vi "Write XML Node.vi"(6 "attributes":T1[](array[typedef]), 8 "error in (no error)":errorcluster, 9 "body":string, 10 "node":string, 11 "initial string":string) -> (0 "error out":errorcluster, 3 "resulting string":string)   [LabVIEW 2020, in "XMLGen.lvlib"]
uses:
  <vilib>/AppBuilder/Engine/WebServiceDescription/XMLGen/XMLGen.lvlib
  <vilib>/AppBuilder/Engine/WebServiceDescription/XMLGen/ValuePair.ctl
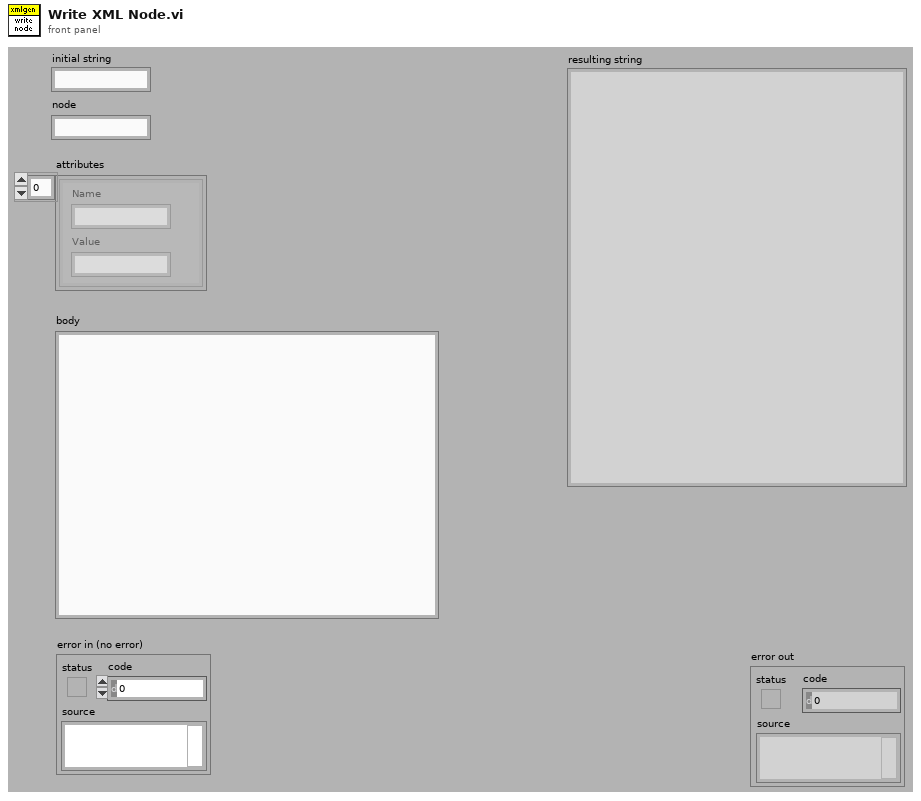
[diagram p1: front panel]
types:
  T1 = typedef "XMLGen.lvlib/ValuePair.ctl" = cluster{"Name":string, "Value":string}
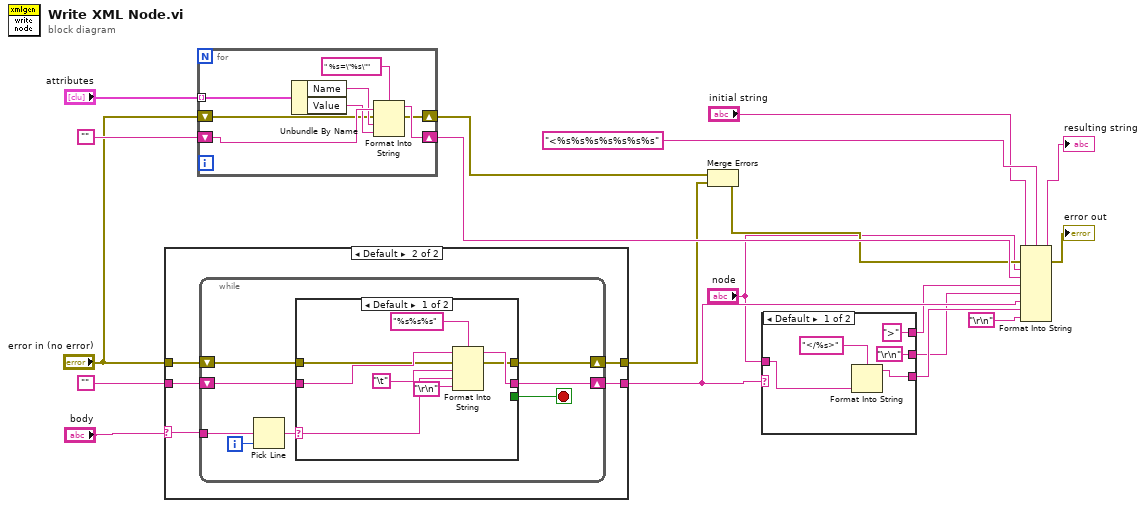
[diagram p0: block diagram]
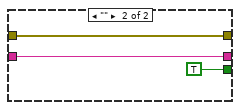
[diagram p3: hidden frame]
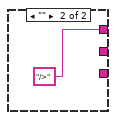
[diagram p4: hidden frame]
diagram:
  n1 = case shown="Default" "body" {
    selector: "body" -> [w21 w22]
    tunnel: "" -> [_ w26]
    tunnel: "error in (no error)" -> [w20 w25]
    tunnel: [w20 w24] -> w12
    tunnel: [w21 w23] -> w5
    frame "" {
    }
    frame Default {
      n2 = while {
        shift-right: [w29] -> w23
        shift-left: w26 -> [w30]
        tunnel: w22 -> [w33]
        shift-right: [w27] -> w24
        shift-left: w25 -> [w28]
        i -> [w34]
        stop <- w31 stop-if-true
        n3 = Pick Line(multi-line string=w33, line index=w34) -> (output string=w32:string)  [unwired: 1 out]
        n4 = case shown="Default" w32 {
          selector: w32 -> [w41 _]
          tunnel: [_ TRUE] -> w31
          tunnel: [w38 w45] -> w29
          tunnel: w30 -> [w42 w45]
          tunnel: w28 -> [w37 w44]
          tunnel: [w36 w44] -> w27
          frame Default {
            n5 = Format Into String(format string="%s%s%s", initial string=w42, error in=w37, "\t", w41, "\r\n") -> (resulting string=w38:string, error out=w36:errorcluster)
          }
          frame "" {
          }
        }
      }
    }
  }
  n6 = for {
    tunnel: "attributes" -> [w51] mode=indexing
    shift-right: [w48] -> w16
    shift-left: "" -> [w53]
    shift-right: [w46] -> w13
    shift-left: "error in (no error)" -> [w47]
    n7 = Unbundle By Name(w51) -> ("Name"=w50:string, "Value"=w49:string)
    n8 = Format Into String(format string=" %s=\"%s\"", initial string=w53, error in=w47, w50, w49) -> (resulting string=w48:string, error out=w46:errorcluster)
  }
  n9 = Merge Errors(w13, w12) -> (w11:errorcluster)
  n10 = case shown="Default" w5 {
    tunnel: [w58 _] -> w6
    tunnel: "node" -> [w56 _]
    tunnel: [">" "/>"] -> w2
    tunnel: ["\r\n" _] -> w1
    frame Default {
      n11 = Format Into String(format string="</%s>", w56) -> (resulting string=w58:string)  [unwired: 2 in, 1 out]
    }
    frame "" {
    }
  }
  n12 = Format Into String(format string="<%s%s%s%s%s%s%s", initial string="initial string", error in=w11, "node", w16, w2, w1, w5, w6, "\r\n") -> (resulting string=→"resulting string":string, error out=→"error out":errorcluster)
